vi "Non Delay Scheduler For Tardiness.vi"(8 "Number of  Jobs":i32=4, 9 "Number of Machines":i32=4, 10 "Processing Times":u16[][](array[numeric])=[[34, 15, 38, 95], [2, 89, 19, 7], [54, 70, 28, 34], [61, 9, 87, 29]], 11 "Schedule":u16[](array[numeric])=[12, 0, 7, 2, 6, 3, 13, 5, 1, 4, 14, 11, 10, 15, 8, 9]) -> (0 "Scheduled Jobs Order":u16[](array[numeric]), 1 "Job Completion Times":u16[](array[numeric]), 2 "Completion Times":u16[][](array[numeric]), 3 "Start Times":u16[][](array[numeric]), 4 "Machine Completion Times":u16[](array[numeric]))   [LabVIEW 2013, in "GanntChart.lvclass"]
uses:
  GanntChart.lvclass
panel:
  out "Indices":i32[](array[numeric])
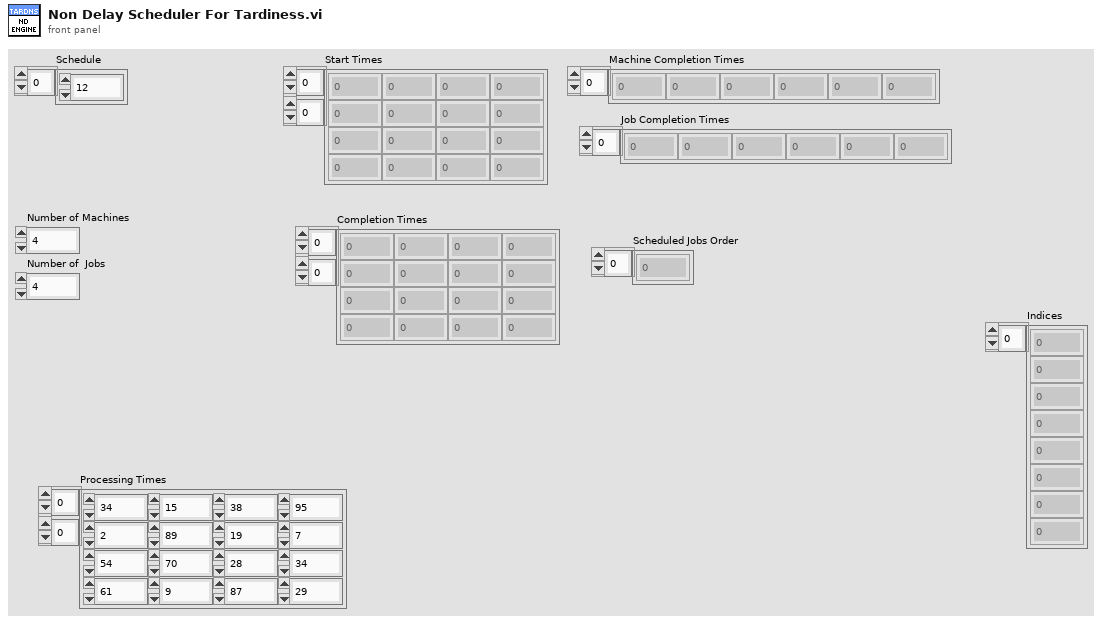
[diagram p1: front panel]
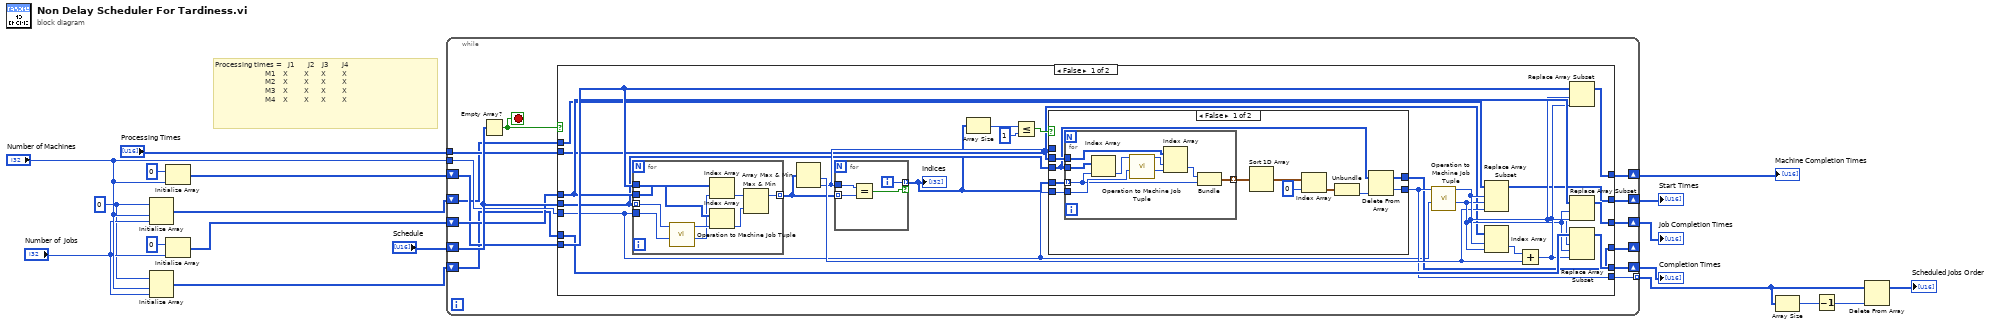
[diagram p0: block diagram]
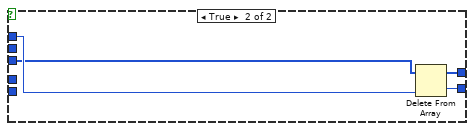
[diagram p2: hidden frame]
diagram:
  w3 = u16 0 ("element")
  # "Processing tImes =   J1       J2    J3       J4   \n                         M1    X        X      X        X\n                         M2    X        X      X        X\n                         M3    X        X      X        X\n                         M4    X        X      X        X"
  n1 = Initialize Array(w3, "Number of Machines", "Number of  Jobs") -> (w2:u16[][])
  n2 = Initialize Array(w3, "Number of Machines", "Number of  Jobs") -> (w14:u16[][])
  n3 = Initialize Array(u16 0 ("element"), "Number of Machines") -> (w16:u16[])
  n4 = Initialize Array(u16 0 ("element"), "Number of  Jobs") -> (w17:u16[])
  n5 = while {
    shift-right: [w25] -> _
    shift-left: "Schedule" -> [w32]
    tunnel: "Number of Machines" -> [w31]
    shift-right: [w28] -> w12
    shift-left: w17 -> [w30]
    shift-right: [w27] -> w11
    shift-left: w16 -> [w29]
    shift-right: [w23] -> w13
    shift-left: w14 -> [w24]
    tunnel: "Processing Times" -> [w26]
    tunnel: [w22] -> w9 mode=indexing
    shift-right: [w20] -> w1
    shift-left: w2 -> [w21]
    stop <- w33 stop-if-true
    n6 = Empty Array?(array=w32) -> (empty?=w33:bool)
    n7 = case shown="False" w33 {
      tunnel: w32 -> [w39 w97]
      tunnel: w31 -> [w34 _]
      tunnel: w30 -> [w56 w99]
      tunnel: w29 -> [w57 w98]
      tunnel: [w55 w99] -> w28
      tunnel: [w54 w98] -> w27
      tunnel: w26 -> [w36 _]
      tunnel: [w37 w97] -> w25
      tunnel: w24 -> [w53 w96]
      tunnel: [w52 w96] -> w23
      tunnel: [w38 _] -> w22
      tunnel: w21 -> [w49 w95]
      tunnel: [w45 w95] -> w20
      frame False {
        n8 = for {
          tunnel: w39 -> [w94] mode=indexing
          tunnel: w34 -> [w93]
          tunnel: w56 -> [w90]
          tunnel: w57 -> [w92]
          tunnel: [w86] -> w44 mode=indexing
          n9 = call "Operation to Machine Job Tuple.vi"("Number of Machines"=w93, "Operation Number"=w94) -> ("Job No"=w89:i32, "Machine No"=w91:i32)  [unwired: 8 in]
          n10 = Index Array(array=w90, index=w89) -> (element=w88:u16)
          n11 = Index Array(array=w92, index=w91) -> (element=w87:u16)
          n12 = Max & Min(x=w88, y=w87) -> (max(x,y)=w86:u16)  [unwired: 1 out]
        }
        n13 = Array Max & Min(array=w44) -> (min value=w46:u16, min index (indices)=w40:i32)  [unwired: 2 out]
        n14 = for {
          tunnel: w44 -> [w85] mode=indexing
          tunnel: w40 -> [w84]
          tunnel: [w83] -> w35 mode=indexing if=w82
          i -> [w83]
          n15 = Equal?(x=w84, y=w85) -> (x = y?=w82:bool)
        }
        "Indices" <- w35
        n16 = Array Size(array=w35) -> (size(s)=w43:i32)
        n17 = Less Or Equal?(x=w43, y=1) -> (x <= y?=w41:bool)
        n18 = case shown="False" w41 {
          tunnel: w40 -> [_ w81]
          tunnel: w39 -> [w61 w80]
          tunnel: [w58 w79] -> w37
          tunnel: [w59 w78] -> w38
          tunnel: w36 -> [w66 _]
          tunnel: w35 -> [w68 _]
          tunnel: w34 -> [w67 _]
          frame False {
            n19 = for {
              tunnel: w68 -> [w71] mode=indexing
              tunnel: w61 -> [w77]
              tunnel: w67 -> [w76]
              tunnel: w66 -> [w75]
              tunnel: [w70] -> w65 mode=indexing
              n20 = Index Array(array=w77, index=w71) -> (element=w69:u16)
              n21 = call "Operation to Machine Job Tuple.vi"("Number of Machines"=w76, "Operation Number"=w69) -> ("Job No"=w73:i32, "Machine No"=w74:i32)  [unwired: 8 in]
              n22 = Index Array(array=w75, index (row)=w74, index (col)=w73) -> (element=w72:u16)
              n23 = Bundle("Numeric"=w72, w71) -> (w70:cluster{"Numeric":u16, i32})  [unwired: 1 in]
            }
            n24 = Sort 1D Array(array=w65) -> (sorted array=w64:cluster{"Numeric":u16, i32}[])
            n25 = Index Array(array=w64, index=0) -> (element=w62:cluster{"Numeric":u16, i32})
            n26 = Unbundle(w62) -> (w60:i32)  [unwired: 1 out]
            n27 = Delete From Array(array=w61, index=w60) -> (deleted portion=w59:u16, array with subset deleted=w58:u16[])  [unwired: 1 in]
          }
          frame True {
            n28 = Delete From Array(array=w80, index=w81) -> (deleted portion=w78:u16, array with subset deleted=w79:u16[])  [unwired: 1 in]
          }
        }
        n29 = call "Operation to Machine Job Tuple.vi"("Number of Machines"=w34, "Operation Number"=w38) -> ("Job No"=w47:i32, "Machine No"=w48:i32)  [unwired: 8 in]
        n30 = Replace Array Subset(array=w49, new element=w46, index (row)=w48, index (col)=w47) -> (w45:u16[][])
        n31 = Index Array(array=w36, index (row)=w48, index (col)=w47) -> (element=w51:u16)
        n32 = Add(x=w51, y=w46) -> (x+y=w50:u16)
        n33 = Replace Array Subset(array=w57, new element=w50, index=w48) -> (w54:u16[])
        n34 = Replace Array Subset(array=w56, new element=w50, index=w47) -> (w55:u16[])
        n35 = Replace Array Subset(array=w53, new element=w50, index (row)=w48, index (col)=w47) -> (w52:u16[][])
      }
      frame True {
      }
    }
  }
  "Completion Times" <- w13
  "Job Completion Times" <- w12
  "Machine Completion Times" <- w11
  "Start Times" <- w1
  n36 = Array Size(array=w9) -> (size(s)=w8:i32)
  n37 = Decrement(x=w8) -> (x-1=w7:i32)
  n38 = Delete From Array(array=w9, index=w7) -> (array with subset deleted=→"Scheduled Jobs Order":u16[])  [unwired: 1 in, 1 out]
